vi "OAT Digital Tacho Process (N Tachos).vi"(0 "digital tacho info":T3[](array[typedef]), 2 "reset? (F)":bool, 7 "pulse/revolution (1)":i32[](array[numeric]), 9 "signal duration [s]":dbl[](array[numeric]) format="%0.2f", 11 "error in (no error)":errorcluster) -> (4 "speed profiles":T2[](array[typedef]) {"speed [RPM]" format="%.2f"; "time [s]" format="%.2f"}, 8 "speed position info":T1[](array[typedef]), 10 "no tacho?":bool[](array[boolean]), 15 "error out":errorcluster)   [LabVIEW 2017, in "SoundVib_TachProcess.lvlib"]
doc: "Locates tachometer pulse positions in the digital tachometer signal and calculates the rotational speed of a device. Wire data to the <B>digital tacho info</B> input to determine the polymorphic instance to use or manually select the instance."
uses:
  <vilib>/addons/Sound and Vibration/Order Analysis/Tach Process/SoundVib_TachProcess.lvlib
  <vilib>/addons/Sound and Vibration/Order Analysis/Tach Process/SubVIs/digital tach info.ctl
  <vilib>/addons/Sound and Vibration/Order Analysis/Tach Process/SubVIs/speed profile.ctl
  <vilib>/addons/Sound and Vibration/Order Analysis/Misc/OAT Position Info.ctl
  <vilib>/addons/Sound and Vibration/Order Analysis/Tach Process/SubVIs/oa_Get Angular Speed (N Tach).vi
  <vilib>/addons/Sound and Vibration/Order Analysis/Tach Process/SubVIs/oa_Process Counter Data (N Tach).vi
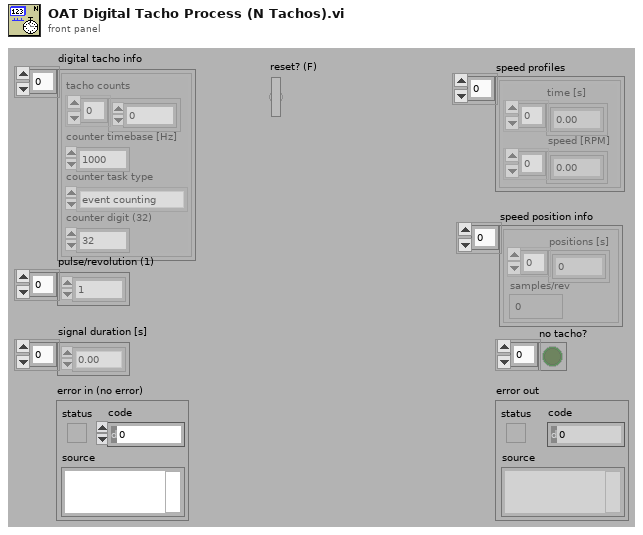
[diagram p1: front panel]
types:
  T1 = typedef "OAT Position Info.ctl" = cluster{"positions [s]":dbl[], "samples/rev":dbl}
  T2 = typedef "SoundVib_TachProcess.lvlib/speed profile.ctl" = cluster{"time [s]":dbl[], "speed [RPM]":dbl[]}
  T3 = typedef "SoundVib_TachProcess.lvlib/digital tach info.ctl" = cluster{"tacho counts":i64[], "counter timebase [Hz]":dbl, "counter task type":enum16{"period measurement", "event counting"}, "counter digit (32)":i32}
  T4 = cluster{"pulse positions [s]":dbl[], "counter timebase [Hz]":dbl, "counter task type":enum16{"period measurement", "event counting"}, "counter digit":i32}[]
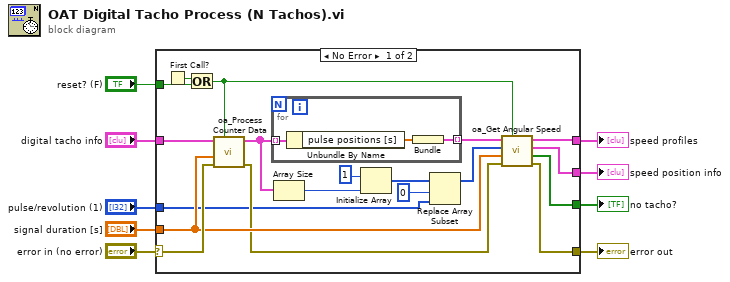
[diagram p0: block diagram]
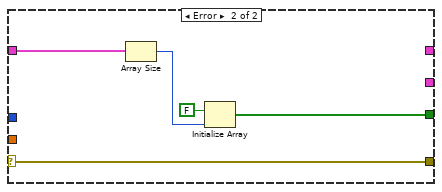
[diagram p2: hidden frame]
diagram:
  n1 = case shown="No Error" "error in (no error)" {
    selector: "error in (no error)" -> [w27 w36]
    tunnel: [w11 w36] -> w9
    tunnel: "digital tacho info" -> [w28 w35]
    tunnel: [w14 _] -> w7
    tunnel: [w12 w32] -> w6
    tunnel: "pulse/revolution (1)" -> [w10 _]
    tunnel: "signal duration [s]" -> [w16 _]
    tunnel: [w13 _] -> w2
    tunnel: "reset? (F)" -> [w25 _]
    frame No Error {
      n2 = First Call?() -> (First Call?: T/F=w26:bool)
      n3 = Or(x=w26, y=w25) -> (x .or. y?=w17:bool)
      n4 = call-poly <vilib>:"oa_Process Counter Data.vi"("reset?(True)"=w17, "error in (no error)"=w27, "vibration data durations [s]"=w16, "digital tach info"=w28) -> ("error out (no error)"=w15:errorcluster, "digital tach info out (DBL)"=w18:T4)  [unwired: 6 in]
      n5 = for {
        tunnel: w18 -> [w31] mode=indexing
        tunnel: [w30] -> w21 mode=indexing
        n6 = Unbundle By Name(w31) -> ("pulse positions [s]"=w29:dbl[])
        n7 = Bundle("pulse positions [s]"=w29) -> (w30:cluster{"pulse positions [s]":dbl[]})  [unwired: 1 in]
      }
      n8 = Array Size(array=w18) -> (size(s)=w19:i32)
      n9 = Initialize Array(1 ("element"), w19) -> (w22:i32[])
      n10 = Replace Array Subset(array=w22, new element=w10, index=0) -> (w20:i32[])
      n11 = call-poly <vilib>:"oa_Get Angular Speed.vi"("reset? (True)"=w17, "error in (no error)"=w15, "durations"=w16, "pulse/revolution (1)"=w20, "pulse position [s]"=w21) -> ("error out"=w11:errorcluster, "No Tach? (False)"=w12:bool[], "speed position info"=w13:T1[], "speed profile"=w14:T2[])  [unwired: 3 in]
    }
    frame Error {
      n12 = Array Size(array=w35) -> (size(s)=w34:i32)
      n13 = Initialize Array(FALSE, w34) -> (w32:bool[])
    }
  }
  "error out" <- w9
  "speed profiles" <- w7
  "no tacho?" <- w6
  "speed position info" <- w2
